vi "niFpgaPID_PDMemoryWrite.vi"(0 "data memory in":refnum<k21>="Data", 1 "channel (0)":u8, 5 "manual memory in":refnum<k21>="Manual", 11 "state in":T1, 12 "parameters in":T2) -> ()   [LabVIEW 2017]
uses:
  <vilib>/rvi/Analysis/control/PID/Typedef/niFpgaPID_PDParameters.ctl
  <vilib>/rvi/Analysis/control/PID/Typedef/niFpgaPID_PDState.ctl
  <vilib>/rvi/Analysis/control/PID/Typedef/niFpgaPID_PIMemoryItem.ctl
  <vilib>/Platform/TimedLoop/XDataNode/timing_clust.ctl
  <vilib>/Platform/TimedLoop/XDataNode/nitl_modes.ctl
  <vilib>/Platform/TimedLoop/XDataNode/wakeup.ctl
  <vilib>/rvi/Emulation/niFpgaSctlEmulationGetInTimedLoop.vi
  <vilib>/Utility/error.llb/Clear Errors.vi
  <vilib>/rvi/DataTransferAndStorage/Container/Common/niFpgaContainerExecOnDevCompGetState.vi
  <vilib>/rvi/Emulation/niFpgaEmulationIsFPGAContextNoSignature.vi
  <vilib>/rvi/DataTransferAndStorage/Container/Common/niFpgaContainerGetUniqueNameForEmu.vi
  <vilib>/rvi/Emulation/niFpgaProcessEmulError.vi
  <vilib>/rvi/errors/nirviReportUnexpectedCaseInternalError (U32).vi
  <vilib>/rvi/Memory/Memory_Emulation/niFpgaMemoryEmulationCacheClearOnFirstRun.vi
  <vilib>/rvi/Memory/Memory_Emulation/nirvimemoryEmulationManagerCache_MakeExclusive.vi
  <vilib>/rvi/Memory/Memory_Emulation/niFpgaMemoryEmulationValidateCache.vi
  <vilib>/rvi/Memory/Memory_Emulation/nirvimemoryEmulationManagerCache_InsertValue.vi
  <vilib>/rvi/Memory/Memory_Emulation/nirvimemoryEmulationManagerCache_ReleaseExclusive.vi
  <vilib>/rvi/Memory/Memory_Emulation/nirvimemoryEmulationManagerCache_GetValue.vi
  <vilib>/rvi/Memory/Memory_Emulation/nirvimemoryEmulationManagerCache_SetValue.vi
  <vilib>/rvi/Emulation/niFpgaSctlEmulationResourceMgr.vi
  <vilib>/Platform/TimedLoop/XDataNode/XDataNode.xnode
  <vilib>/rvi/DataTransferAndStorage/Container/XNode/niFpgaContainer.xnode
  <vilib>/rvi/Memory/Memory_Emulation/niFpgaMemoryEmulationRefIn.vi
  <vilib>/Platform/TimedLoop/XDataNode/XDNodeRunTimeDep.lvlib
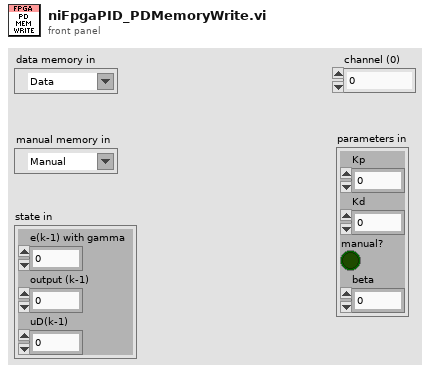
[diagram p1: front panel]
types:
  T1 = typedef "niFpgaPID_PDState.ctl" = cluster{"e(k-1) with gamma":sgl, "output (k-1)":sgl, "uD(k-1)":sgl}
  T2 = typedef "niFpgaPID_PDParameters.ctl" = cluster{"Kp":sgl, "Kd":sgl, "manual?":bool, "beta":sgl}
  T3 = typedef "niFpgaPID_PIMemoryItem.ctl" = cluster{"data 1":sgl, "data 2":sgl, "data 3":sgl}
  T4 = typedef "XDNodeRunTimeDep.lvlib/timing_clust.ctl" = cluster{"Expected End [f-1]":u64, "Actual End [f-1]":u64, "Finished Late? [f-1]":bool, "Expected End [i-1]":u64, "Actual End [i-1]":u64, "Finished Late? [i-1]":bool, "Expected Start [i]":u64, "Actual Start [i]":u64, "Expected Start [f]":u64, "Actual Start [f]":u64, "Source Name":string, "Structure Name":string, "Period":i64, "Deadline":i64, "Offset":i64, "Start":i64, "Priority":i32, "Timeout":i32, "Mode":T5, "Wakeup Reason":T6, "Error":errorcluster, "Source Type":string, "Secondary Source Type":string, "Global End Time":u64, "Global Start Time":u64, "Frame Duration":u64, "Iteration Duration":u64, "Assigned CPU":i32, "I/O Scan Engine Mode":u32}
  T5 = typedef "XDNodeRunTimeDep.lvlib/nitl_modes.ctl" = enum32{"No Change", "Process missed periods, maintain original phase", "Discard missed periods, maintain original phase", "Process missed periods, ignore original phase", "Discard missed periods, ignore original phase"}
  T6 = typedef "XDNodeRunTimeDep.lvlib/wakeup.ctl" = enum32{"Normal", "Aborted", "Asynchronous wakeup", "Timing source error", "Timed loop error", "Timeout"}
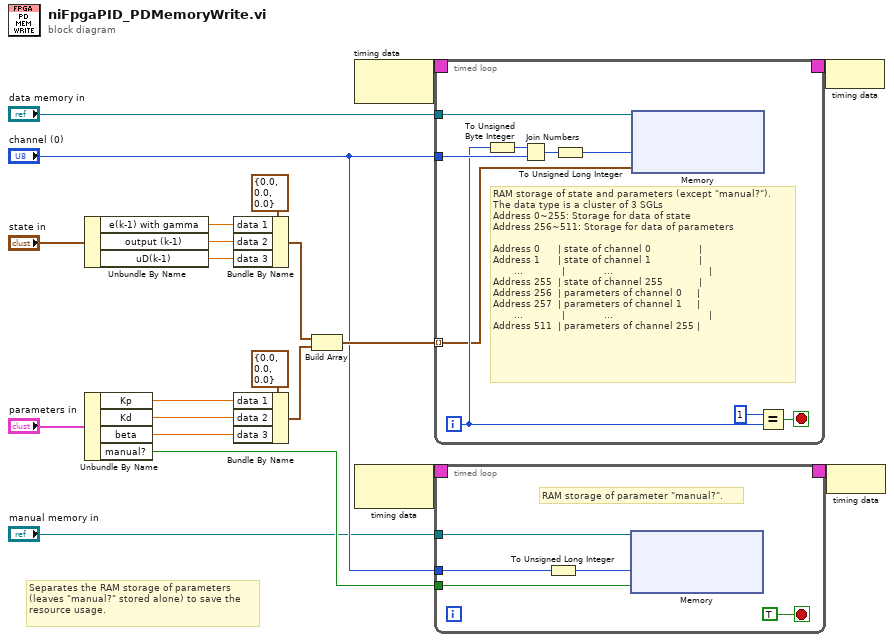
[diagram p0: block diagram]
diagram:
  # "Separates the RAM storage of parameters\n(leaves \"manual?\" stored alone) to save the \nresource usage."
  n1 = Unbundle By Name("state in") -> ("e(k-1) with gamma"=w16:sgl, "output (k-1)"=w14:sgl, "uD(k-1)"=w15:sgl)
  n2 = Unbundle By Name("parameters in") -> ("Kp"=w13:sgl, "Kd"=w12:sgl, "beta"=w9:sgl, "manual?"=w6:bool)
  n3 = Bundle By Name(cluster=T3 {"data 1"=0.0, "data 2"=0.0, "data 3"=0.0} ("PID state and parameters"), "data 1"=w16, "data 2"=w14, "data 3"=w15) -> (w19:T3)
  n4 = Bundle By Name(cluster=T3 {"data 1"=0.0, "data 2"=0.0, "data 3"=0.0} ("PI state and parameters"), "data 1"=w13, "data 2"=w12, "data 3"=w9) -> (w18:T3)
  n5 = Build Array(w19, w18) -> (w17:T3[])
  n6 = node-c288() -> (w21:T4)  [unwired: 1 in]
  n7 = node-c288() -> (w8:T4)  [unwired: 1 in]
  n8 = timed-loop {
    timing: w21 -> [_]
    timing-out: [_] -> w20
    tunnel: "data memory in" -> [w24]
    tunnel: "channel (0)" -> [w28]
    tunnel: w17 -> [w22] mode=indexing
    i -> [w27]
    stop <- w30 stop-if-true
    # "RAM storage of state and parameters (except \"manual?\").\nThe data type is a cluster of 3 SGLs \nAddress 0~255: Storage for data of state\nAddress 256~511: Storage for data of parameters\n                                                                         \nAddress 0      | state of channel 0                | \nAddress 1      | state of channel 1                | \n       ...             |             ...                                |\nAddress 255  | state of channel 255            | \nAddress 256  | parameters of channel 0     | \nAddress 257  | parameters of channel 1     | \n       ...             |             ...                                |\nAddress 511  | parameters of channel 255 |"
    n9 = To Unsigned Byte Integer(number=w27) -> (unsigned 8bit integer=w26:u8)
    n10 = Join Numbers(hi=w26, lo=w28) -> ((hi.lo)=w29:u16)
    n11 = To Unsigned Long Integer(number=w29) -> (unsigned 32bit integer=w23:u32)
    n12 = xnode "Memory"("Address"=w23, "Data"=w22, "Memory In"=w24) -> ()  [unwired: 1 out]
    n13 = Equal?(x=1, y=w27) -> (x = y?=w30:bool)
  }
  n14 = timed-loop {
    timing: w8 -> [_]
    timing-out: [_] -> w7
    tunnel: "manual memory in" -> [w35]
    tunnel: w6 -> [w34]
    tunnel: "channel (0)" -> [w37]
    stop <- TRUE stop-if-true
    # "RAM storage of parameter \"manual?\"."
    n15 = To Unsigned Long Integer(number=w37) -> (unsigned 32bit integer=w33:u32)
    n16 = xnode "Memory"("Address"=w33, "Data"=w34, "Memory In"=w35) -> ()  [unwired: 1 out]
  }
  n17 = node-c288(w20) -> ()
  n18 = node-c288(w7) -> ()
